vi "CRC_Modbus.vi"(11 "IN":string) -> (1 "CRC":string, 2 "Out":string, 3 "输出变量":u16 format="%x")   [LabVIEW 2013]
panel:
  out "长度":i32
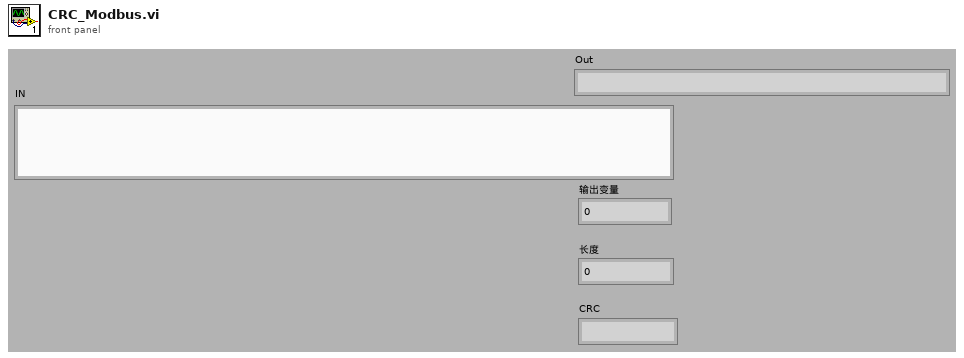
[diagram p1: front panel]
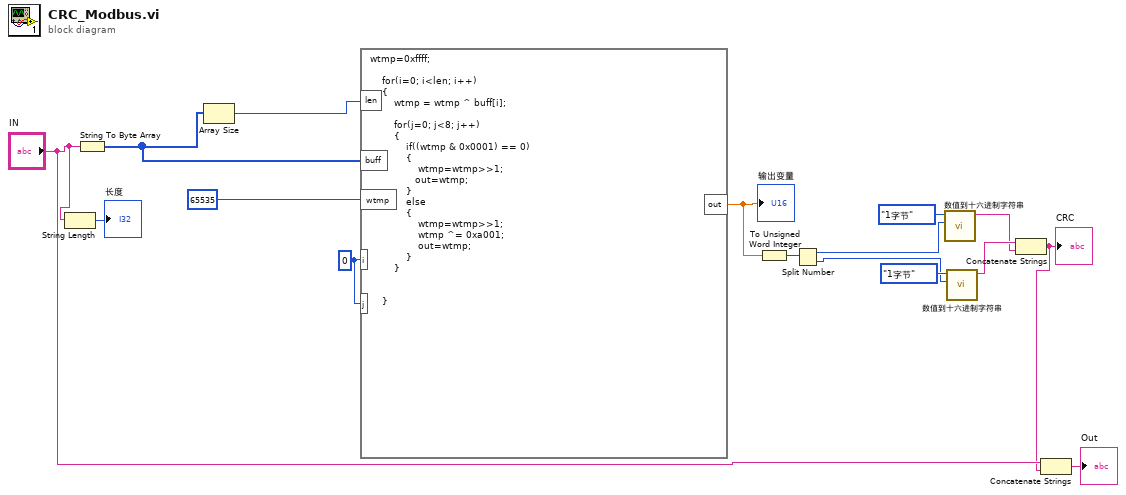
[diagram p0: block diagram]
diagram:
  w15 = u8 0 ("输入变量")
  n1 = String Length(string="IN") -> (length=→"长度":i32)
  n2 = String To Byte Array(string="IN") -> (unsigned byte array=w14:u8[])
  n3 = Array Size(array=w14) -> (size(s)=w12:i32)
  n4 = formula code="wtmp=0xffff;\n\n    for(i=0; i<len; i++) \n    {\n        wtmp = wtmp ^ buff[i];\n        \n        for(j=0; j<8; j++) \n        {\n            if((wtmp & 0x0001) == 0)\n            {\n                wtmp=wtmp>>1;  \n               out=wtmp;\n            } \n            else\n            {\n                wtmp=wtmp>>1;\n                wtmp ^= 0xa001;   \n                out=wtmp;\n            }\n        }\n        \n        \n    }"("buff"=w14, "wtmp"=u16 65535 ("数值"), "i"=w15, "j"=w15, "len"=w12) -> ("out"=w11:dbl)
  "输出变量" <- w11
  n5 = To Unsigned Word Integer(number=w11) -> (unsigned 16bit integer=w10:u16)
  n6 = Split Number(x=w10) -> (hi(x)=w8:u8, lo(x)=w6:u8)
  n7 = call "数值到十六进制字符串.vi"("Numeric"=w8, "转换字节数"=enum16{"1字节", "2字节", "4字节", "3字节"}."1字节") -> ("转换结果"=w4:string)  [unwired: 8 in, 1 out]
  n8 = call "数值到十六进制字符串.vi"("Numeric"=w6, "转换字节数"=enum16{"1字节", "2字节", "4字节", "3字节"}."1字节") -> ("转换结果"=w5:string)  [unwired: 8 in, 1 out]
  n9 = Concatenate Strings(w5, w4) -> (w2:string)
  "CRC" <- w2
  n10 = Concatenate Strings("IN", w2) -> (→"Out":string)
